vi "CRIS responder 2.vi"() -> ()   [LabVIEW 2013]
panel:
  out "isOK":bool
  out "waveSet":dbl
  out "isNew":bool
  out "waveReadback":dbl
  in  "Stop":bool
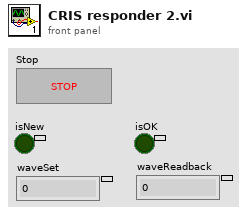
[diagram p1: front panel]
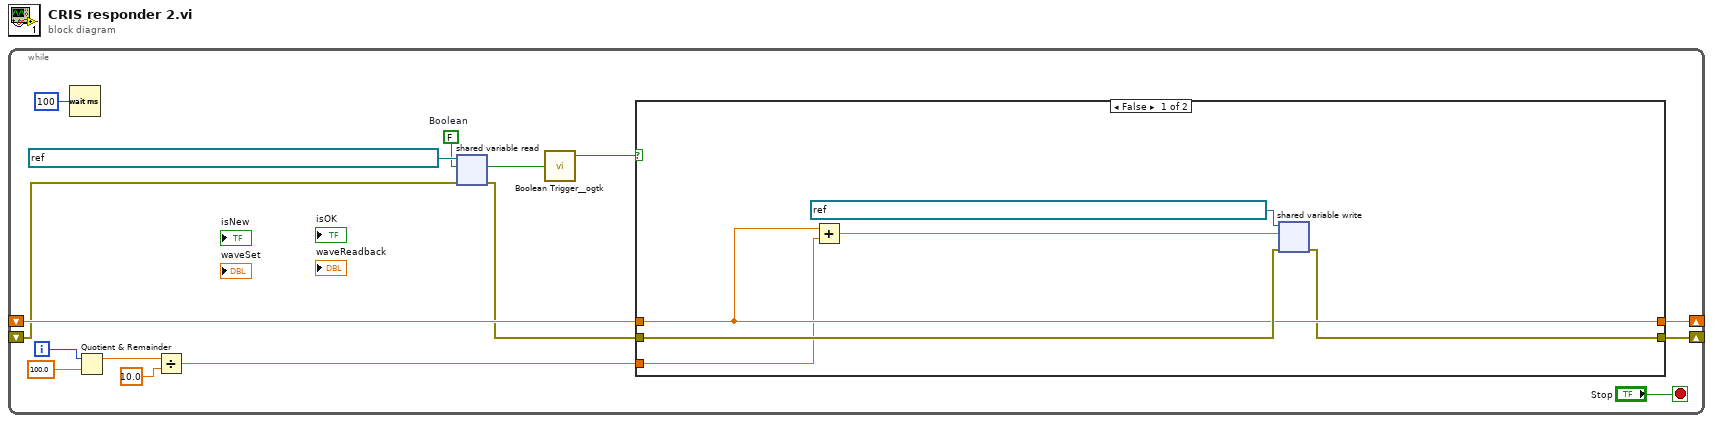
[diagram p0: block diagram]
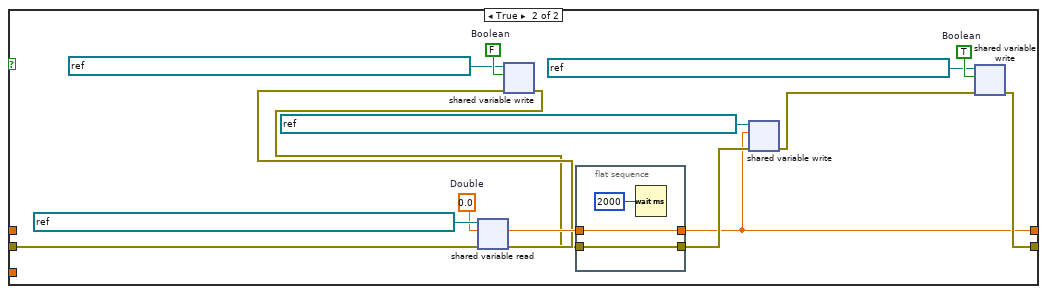
[diagram p2: hidden frame]
diagram:
  n1 = while {
    shift-right: [w10] -> _
    shift-left: _ -> [w9]
    shift-right: [w3] -> _
    shift-left: _ -> [w1]
    i -> [w15]
    stop <- "Stop" stop-if-true
    w7 = FALSE  # Boolean
    n2 = Wait (ms)(milliseconds to wait=u32 100) -> ()  [unwired: 1 out]
    n3 = Quotient & Remainder(x=w15, y=100.0) -> (x-y*floor(x/y)=w12:dbl)  [unwired: 1 out]
    n4 = Divide(x=w12, y=10.0) -> (x/y=w11:dbl)
    n5 = shared-variable-read(refnum<k21> "ni.var.psp://localhost/Narrow Band TiSa Scanner Shared Variables/isNew" ("shared variable refnum in"), w1, w7) -> (w2:errorcluster, w5:bool)  [unwired: 2 out]
    n6 = call <userlib>:"Boolean Trigger__ogtk.vi"("Boolean Input"=w5) -> ("Rising Edge"=w4:bool)  [unwired: 1 in, 1 out]
    n7 = case shown="False" w4 {
      tunnel: [w20 w28] -> w10
      tunnel: w11 -> [w19 _]
      tunnel: w9 -> [w20 _]
      tunnel: [w18 w32] -> w3
      tunnel: w2 -> [w21 w27]
      frame False {
        n8 = Add(x=w20, y=w19) -> (x+y=w17:dbl)
        n9 = shared-variable-write(refnum<k21> "ni.var.psp://localhost/Narrow Band TiSa Scanner Shared Variables/waveReadback" ("shared variable refnum in"), w21, w17) -> (w18:errorcluster)  [unwired: 1 out]
      }
      frame True {
        w26 = FALSE  # Boolean
        w34 = TRUE  # Boolean
        w36 = 0.0  # Double
        n10 = shared-variable-read(refnum<k21> "ni.var.psp://localhost/Narrow Band TiSa Scanner Shared Variables/waveSet" ("shared variable refnum in"), w27, w36) -> (w25:errorcluster, w35:dbl)  [unwired: 2 out]
        n11 = shared-variable-write(refnum<k21> "ni.var.psp://localhost/Narrow Band TiSa Scanner Shared Variables/isOK" ("shared variable refnum in"), w25, w26) -> (w24:errorcluster)  [unwired: 1 out]
        n12 = flat-sequence {
          tunnel: [w39] -> w28
          tunnel: w35 -> [w39]
          tunnel: [w38] -> w30
          tunnel: w24 -> [w38]
          frame #0 {
            n13 = Wait (ms)(milliseconds to wait=u32 2000) -> ()  [unwired: 1 out]
          }
        }
        n14 = shared-variable-write(refnum<k21> "ni.var.psp://localhost/Narrow Band TiSa Scanner Shared Variables/waveReadback" ("shared variable refnum in"), w30, w28) -> (w29:errorcluster)  [unwired: 1 out]
        n15 = shared-variable-write(refnum<k21> "ni.var.psp://localhost/Narrow Band TiSa Scanner Shared Variables/isOK" ("shared variable refnum in"), w29, w34) -> (w32:errorcluster)  [unwired: 1 out]
      }
    }
  }
